vi "Fan_Project_3.vi"() -> ()   [LabVIEW 2019]
panel:
  in  "회전":bool
  in  "STOP?":bool
  in  "예약 시스템":timestamp
  in  "발생":bool
  in  "예약ON/OFF":bool
  in  "강도":u32
  in  "정지":bool
  in  "EXIT?":bool
  in  "Exit":bool
  in  "운행모드":T1
  in  "Display":u16(ring)
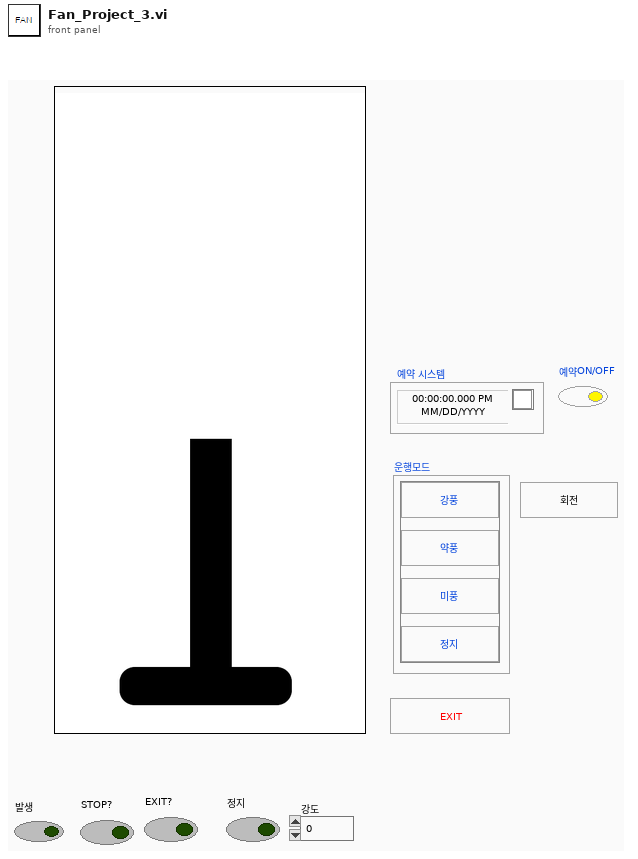
[diagram p1: front panel]
types:
  T1 = cluster{"강풍":bool, "약풍":bool, "미풍":bool, "정지":bool}
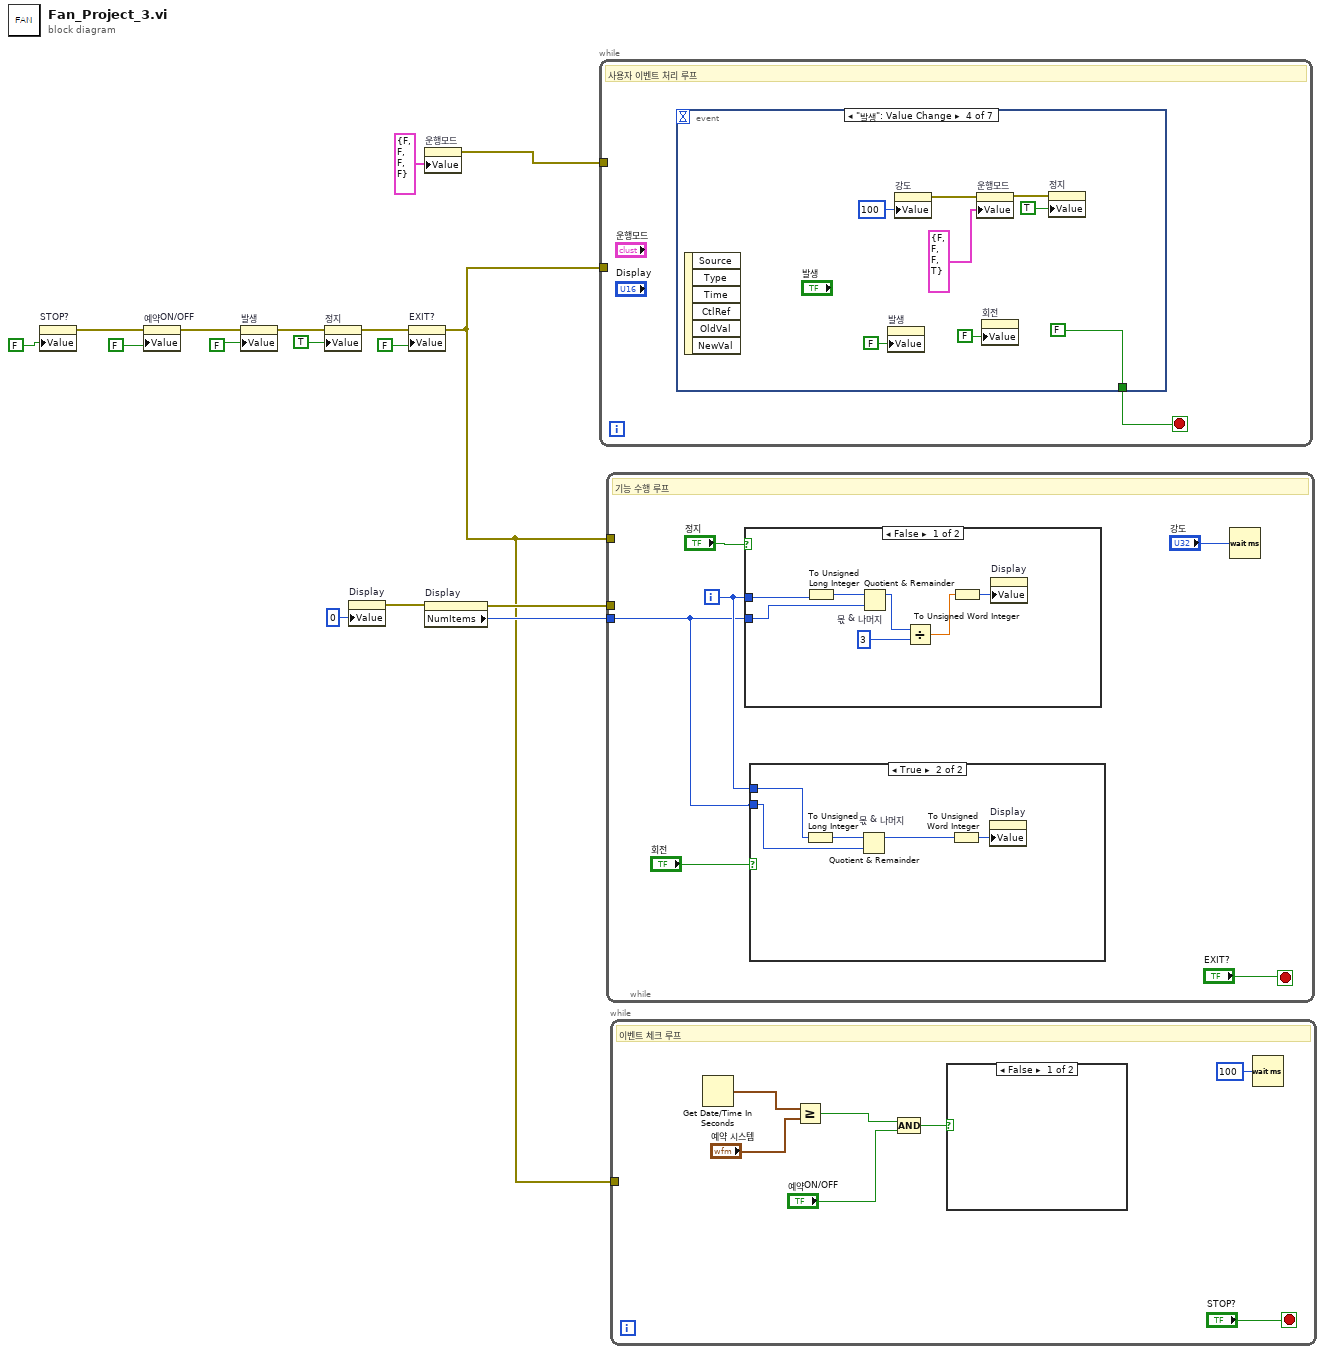
[diagram p0: block diagram]
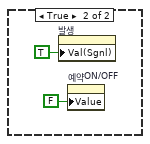
[diagram p2: hidden frame]
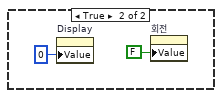
[diagram p4: hidden frame]
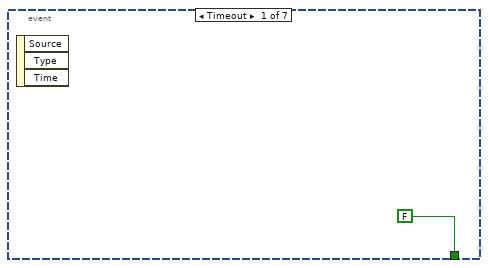
[diagram p5: hidden frame]
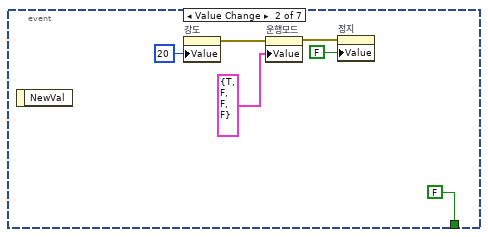
[diagram p6: hidden frame]
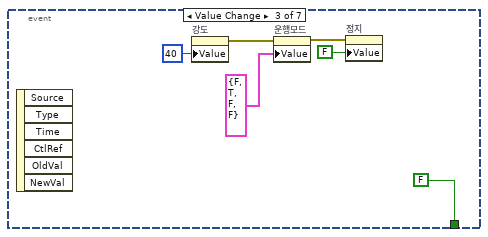
[diagram p7: hidden frame]
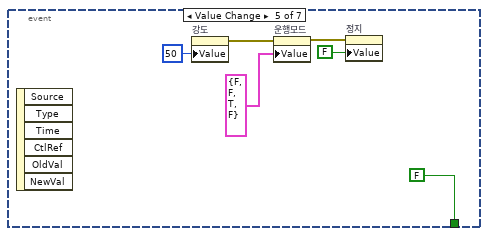
[diagram p8: hidden frame]
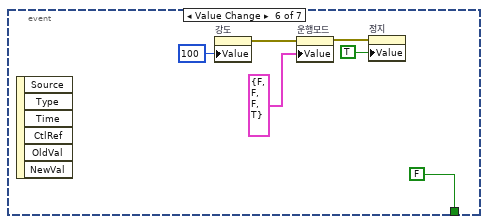
[diagram p9: hidden frame]
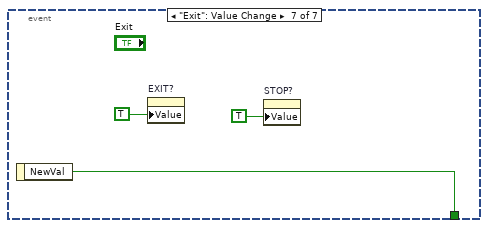
[diagram p10: hidden frame]
diagram:
  n1 = property on="STOP?" class="Bool (strict)"("Value"=FALSE ("STOP?")) -> (error out=w3:errorcluster)  [unwired: 2 in, 1 out]
  n2 = property on="예약ON/OFF" class="Bool (strict)"(error in=w3, "Value"=FALSE ("체크?")) -> (error out=w4:errorcluster)  [unwired: 1 in, 1 out]
  n3 = property on="발생" class="Bool (strict)"(error in=w4, "Value"=FALSE ("발생")) -> (error out=w5:errorcluster)  [unwired: 1 in, 1 out]
  n4 = property on="정지" class="Bool (strict)"(error in=w5, "Value"=TRUE) -> (error out=w8:errorcluster)  [unwired: 1 in, 1 out]
  n5 = property on="Display" class="Ring (strict)"("Value"=u16 0 ("Display")) -> (error out=w11:errorcluster)  [unwired: 2 in, 1 out]
  n6 = property on="EXIT?" class="Bool (strict)"(error in=w8, "Value"=FALSE) -> (error out=w1:errorcluster)  [unwired: 1 in, 1 out]
  n7 = property on="운행모드" class="Clust (strict)"("Value"=T1 {"강풍"=FALSE, "약풍"=FALSE, "미풍"=FALSE, "정지"=FALSE} ("운행모드")) -> (error out=w13:errorcluster)  [unwired: 2 in, 1 out]
  n8 = property on="Display" class="Ring (strict)"(error in=w11) -> (error out=w14:errorcluster, "NumItems"=w15:u32)  [unwired: 1 in, 1 out]
  n9 = while {
    tunnel: w1 -> [_]
    tunnel: w13 -> [_]
    stop <- w17 stop-if-true
    # "사용자 이벤트 처리 루프"
    n10 = event shown="[3] \"발생\": Value Change" {
      selector: _ -> [_ _ _ _ _ _ _]
      dyn-events: _ -> [_ _ _ _ _ _ _]
      timeout: _ -> [_ _ _ _ _ _ _]
      tunnel: [FALSE FALSE FALSE FALSE FALSE FALSE w53] -> w17
      event Timeout {
        n11 = event-data() -> ()  [unwired: 1 in, 3 out]
      }
      event "운행모드.강풍": Value Change {
        n12 = event-data() -> ()  [unwired: 1 in, 1 out]
        n13 = property on="강도" class="DigNum (strict)"("Value"=u32 20 ("쎄기")) -> (error out=w22:errorcluster)  [unwired: 2 in, 1 out]
        n14 = property on="운행모드" class="Clust (strict)"(error in=w22, "Value"=T1 {"강풍"=TRUE, "약풍"=FALSE, "미풍"=FALSE, "정지"=FALSE} ("운행모드")) -> (error out=w23:errorcluster)  [unwired: 1 in, 1 out]
        n15 = property on="정지" class="Bool (strict)"(error in=w23, "Value"=FALSE) -> ()  [unwired: 1 in, 2 out]
      }
      event "운행모드.약풍": Value Change {
        n16 = event-data() -> ()  [unwired: 1 in, 6 out]
        n17 = property on="강도" class="DigNum (strict)"("Value"=u32 40 ("쎄기")) -> (error out=w26:errorcluster)  [unwired: 2 in, 1 out]
        n18 = property on="운행모드" class="Clust (strict)"(error in=w26, "Value"=T1 {"강풍"=FALSE, "약풍"=TRUE, "미풍"=FALSE, "정지"=FALSE} ("운행모드")) -> (error out=w28:errorcluster)  [unwired: 1 in, 1 out]
        n19 = property on="정지" class="Bool (strict)"(error in=w28, "Value"=FALSE) -> ()  [unwired: 1 in, 2 out]
      }
      event "발생": Value Change {
        n20 = event-data() -> ()  [unwired: 1 in, 6 out]
        n21 = property on="발생" class="Bool (strict)"("Value"=FALSE ("발생")) -> ()  [unwired: 2 in, 2 out]
        n22 = property on="강도" class="DigNum (strict)"("Value"=u32 100 ("쎄기")) -> (error out=w37:errorcluster)  [unwired: 2 in, 1 out]
        n23 = property on="운행모드" class="Clust (strict)"(error in=w37, "Value"=T1 {"강풍"=FALSE, "약풍"=FALSE, "미풍"=FALSE, "정지"=TRUE} ("운행모드")) -> (error out=w38:errorcluster)  [unwired: 1 in, 1 out]
        n24 = property on="회전" class="Bool (strict)"("Value"=FALSE ("회전")) -> ()  [unwired: 2 in, 2 out]
        n25 = property on="정지" class="Bool (strict)"(error in=w38, "Value"=TRUE) -> ()  [unwired: 1 in, 2 out]
      }
      event "운행모드.미풍": Value Change {
        n26 = event-data() -> ()  [unwired: 1 in, 6 out]
        n27 = property on="강도" class="DigNum (strict)"("Value"=u32 50 ("쎄기")) -> (error out=w40:errorcluster)  [unwired: 2 in, 1 out]
        n28 = property on="운행모드" class="Clust (strict)"(error in=w40, "Value"=T1 {"강풍"=FALSE, "약풍"=FALSE, "미풍"=TRUE, "정지"=FALSE} ("운행모드")) -> (error out=w42:errorcluster)  [unwired: 1 in, 1 out]
        n29 = property on="정지" class="Bool (strict)"(error in=w42, "Value"=FALSE) -> ()  [unwired: 1 in, 2 out]
      }
      event "운행모드.정지": Value Change {
        n30 = event-data() -> ()  [unwired: 1 in, 6 out]
        n31 = property on="강도" class="DigNum (strict)"("Value"=u32 100 ("쎄기")) -> (error out=w46:errorcluster)  [unwired: 2 in, 1 out]
        n32 = property on="운행모드" class="Clust (strict)"(error in=w46, "Value"=T1 {"강풍"=FALSE, "약풍"=FALSE, "미풍"=FALSE, "정지"=TRUE} ("운행모드")) -> (error out=w49:errorcluster)  [unwired: 1 in, 1 out]
        n33 = property on="정지" class="Bool (strict)"(error in=w49, "Value"=TRUE) -> ()  [unwired: 1 in, 2 out]
      }
      event "Exit": Value Change {
        n34 = event-data() -> ("NewVal"=w53:bool)  [unwired: 1 in]
        n35 = property on="EXIT?" class="Bool (strict)"("Value"=TRUE) -> ()  [unwired: 2 in, 2 out]
        n36 = property on="STOP?" class="Bool (strict)"("Value"=TRUE ("STOP?")) -> ()  [unwired: 2 in, 2 out]
      }
    }
  }
  n37 = while {
    tunnel: w1 -> [_]
    tunnel: w15 -> [w55]
    tunnel: w14 -> [_]
    i -> [w56]
    stop <- "EXIT?" stop-if-true
    # "기능 수행 루프"
    n38 = case shown="False" "정지" {
      tunnel: w55 -> [w68 _]
      tunnel: w56 -> [w69 _]
      frame False {
        n39 = To Unsigned Long Integer(number=w69) -> (unsigned 32bit integer=w71:u32)
        n40 = Quotient & Remainder "몫 & 나머지"(x=w71, y=w68) -> (x-y*floor(x/y)=w67:u32)  [unwired: 1 out]
        n41 = Divide(x=w67, y=u32 3) -> (x/y=w65:dbl)
        n42 = To Unsigned Word Integer(number=w65) -> (unsigned 16bit integer=w70:u16)
        n43 = property on="Display" class="Ring (strict)"("Value"=w70) -> ()  [unwired: 2 in, 2 out]
      }
      frame True {
        n44 = property on="Display" class="Ring (strict)"("Value"=u16 0 ("Display")) -> ()  [unwired: 2 in, 2 out]
        n45 = property on="회전" class="Bool (strict)"("Value"=FALSE ("회전")) -> ()  [unwired: 2 in, 2 out]
      }
    }
    n46 = case shown="True" "회전" {
      tunnel: w56 -> [_ w60]
      tunnel: w55 -> [_ w61]
      frame False {
      }
      frame True {
        n47 = To Unsigned Long Integer(number=w60) -> (unsigned 32bit integer=w63:u32)
        n48 = Quotient & Remainder "몫 & 나머지"(x=w63, y=w61) -> (x-y*floor(x/y)=w62:u32)  [unwired: 1 out]
        n49 = To Unsigned Word Integer(number=w62) -> (unsigned 16bit integer=w64:u16)
        n50 = property on="Display" class="Ring (strict)"("Value"=w64) -> ()  [unwired: 2 in, 2 out]
      }
    }
    n51 = Wait (ms)(milliseconds to wait="강도") -> ()  [unwired: 1 out]
  }
  n52 = while {
    tunnel: w1 -> [_]
    stop <- "STOP?" stop-if-true
    # "이벤트 체크 루프"
    n53 = Get Date/Time In Seconds() -> (seconds since 1Jan1904=w77:timestamp)
    n54 = Greater Or Equal?(x=w77, y="예약 시스템") -> (x >= y?=w75:bool)
    n55 = Compound Arithmetic op=AND(w75, "예약ON/OFF") -> (w79:bool)
    n56 = case shown="False" w79 {
      frame False {
      }
      frame True {
        n57 = property on="발생" class="Bool (strict)"("Val(Sgnl)"=TRUE ("Value (Signaling)")) -> ()  [unwired: 2 in, 2 out]
        n58 = property on="예약ON/OFF" class="Bool (strict)"("Value"=FALSE ("체크?")) -> ()  [unwired: 2 in, 2 out]
      }
    }
    n59 = Wait (ms)(milliseconds to wait=u32 100) -> ()  [unwired: 1 out]
  }
